vi "Close PDF refnum.vi"(1 "Data IN":T1={"Document"=refnum, "Writer"=refnum, "Default Font"=refnum, "Default Font cluster"={"Name"="Helvetica", "Size"=12.0, "Color"=0, "Style"={"Bold"=FALSE, "Italic"=FALSE, "Underline"=FALSE, "Strikeout"=FALSE}}, "Path"=path "", "Unit (default = mm)"=enum."mm", "Paragraphe cluster"={" Aligment"=enum."Select", "Line spacing"=enum."Select"}, "Pages dimensions [ ]"=[], "Captions"={"Image"={"Caption"="", "Separator"="", "Position"=enum."Above"}, "Image counter"=0, "Table"={"Caption"="", "Separator"="", "Position"=enum."Above"}, "Table counter"=0, "Font"={"Name"="", "Size"=-1.0, "Color"=0, "Style"={"Bold"=FALSE, "Italic"=FALSE, "Underline"=FALSE, "Strikeout"=FALSE}}}, "Header"=[], "Footer"=[], "Watermark "={"Show? (F)"=FALSE, "Type"=enum."Text", "Opacity (%)"=10.0, "Rotate(°)"=0.0, "Position"={"Position"=enum."Center (text section)", "X"=0.0, "Y"=0.0}, "Image path"=path "", "Scaled(%)"=100.0, "Image refnum"=refnum, "Text"="CONFIDENTIAL", "Font"={"Name"="", "Size"=-1.0, "Color"=0}, "Font refnum"=refnum, "Alignment"=enum."Center", "Automatic"=FALSE}, "Actual VI name"="", "System Fonts"={"Font name [ ]"=[], "Font and file names [ ]"=[]}} caption="Data") -> (0 "Data OUT":T1={"Document"=refnum, "Writer"=refnum, "Default Font"=refnum, "Default Font cluster"={"Name"="Helvetica", "Size"=12.0, "Color"=0, "Style"={"Bold"=FALSE, "Italic"=FALSE, "Underline"=FALSE, "Strikeout"=FALSE}}, "Path"=path "", "Unit (default = mm)"=enum."mm", "Paragraphe cluster"={" Aligment"=enum."Select", "Line spacing"=enum."Select"}, "Pages dimensions [ ]"=[], "Captions"={"Image"={"Caption"="", "Separator"="", "Position"=enum."Above"}, "Image counter"=0, "Table"={"Caption"="", "Separator"="", "Position"=enum."Above"}, "Table counter"=0, "Font"={"Name"="", "Size"=-1.0, "Color"=0, "Style"={"Bold"=FALSE, "Italic"=FALSE, "Underline"=FALSE, "Strikeout"=FALSE}}}, "Header"=[], "Footer"=[], "Watermark "={"Show? (F)"=FALSE, "Type"=enum."Text", "Opacity (%)"=10.0, "Rotate(°)"=0.0, "Position"={"Position"=enum."Center (text section)", "X"=0.0, "Y"=0.0}, "Image path"=path "", "Scaled(%)"=100.0, "Image refnum"=refnum, "Text"="CONFIDENTIAL", "Font"={"Name"="", "Size"=-1.0, "Color"=0}, "Font refnum"=refnum, "Alignment"=enum."Center", "Automatic"=FALSE}, "Actual VI name"="", "System Fonts"={"Font name [ ]"=[], "Font and file names [ ]"=[]}} caption="Data")   [LabVIEW 2012]
uses:
  PDF Report Data.ctl
  C:/Users/MaxCorp/Documents/TopPerm - Base/DLL/itextsharp.dll
  DLL/itextsharp.dll
  Font cluster.ctl
  Font size.ctl
  Font color.ctl
  Unit.ctl
  Paragraphe cluster.ctl
  Texte alignement.ctl
  Line spacing.ctl
  Page dimensions.ctl
  Page Orientation.ctl
  Image or Table Caption.ctl
  Header Footer [ ].ctl
  Header Footer cluster.ctl
  Header Footer Type.ctl
  Header footer horiz alignment.ctl
  Cell Vertical alignment.ctl
  Page number.ctl
  Header Footer Line.ctl
  Watermark cluster2.ctl
  Watermark Position.ctl
  System Fonts.ctl
  PDF Report.xctl
panel:
  # "X"
  # "Y"
  # "X"
  # "Y"
  # "X"
  # "Y"
  # "X"
  # "Y"
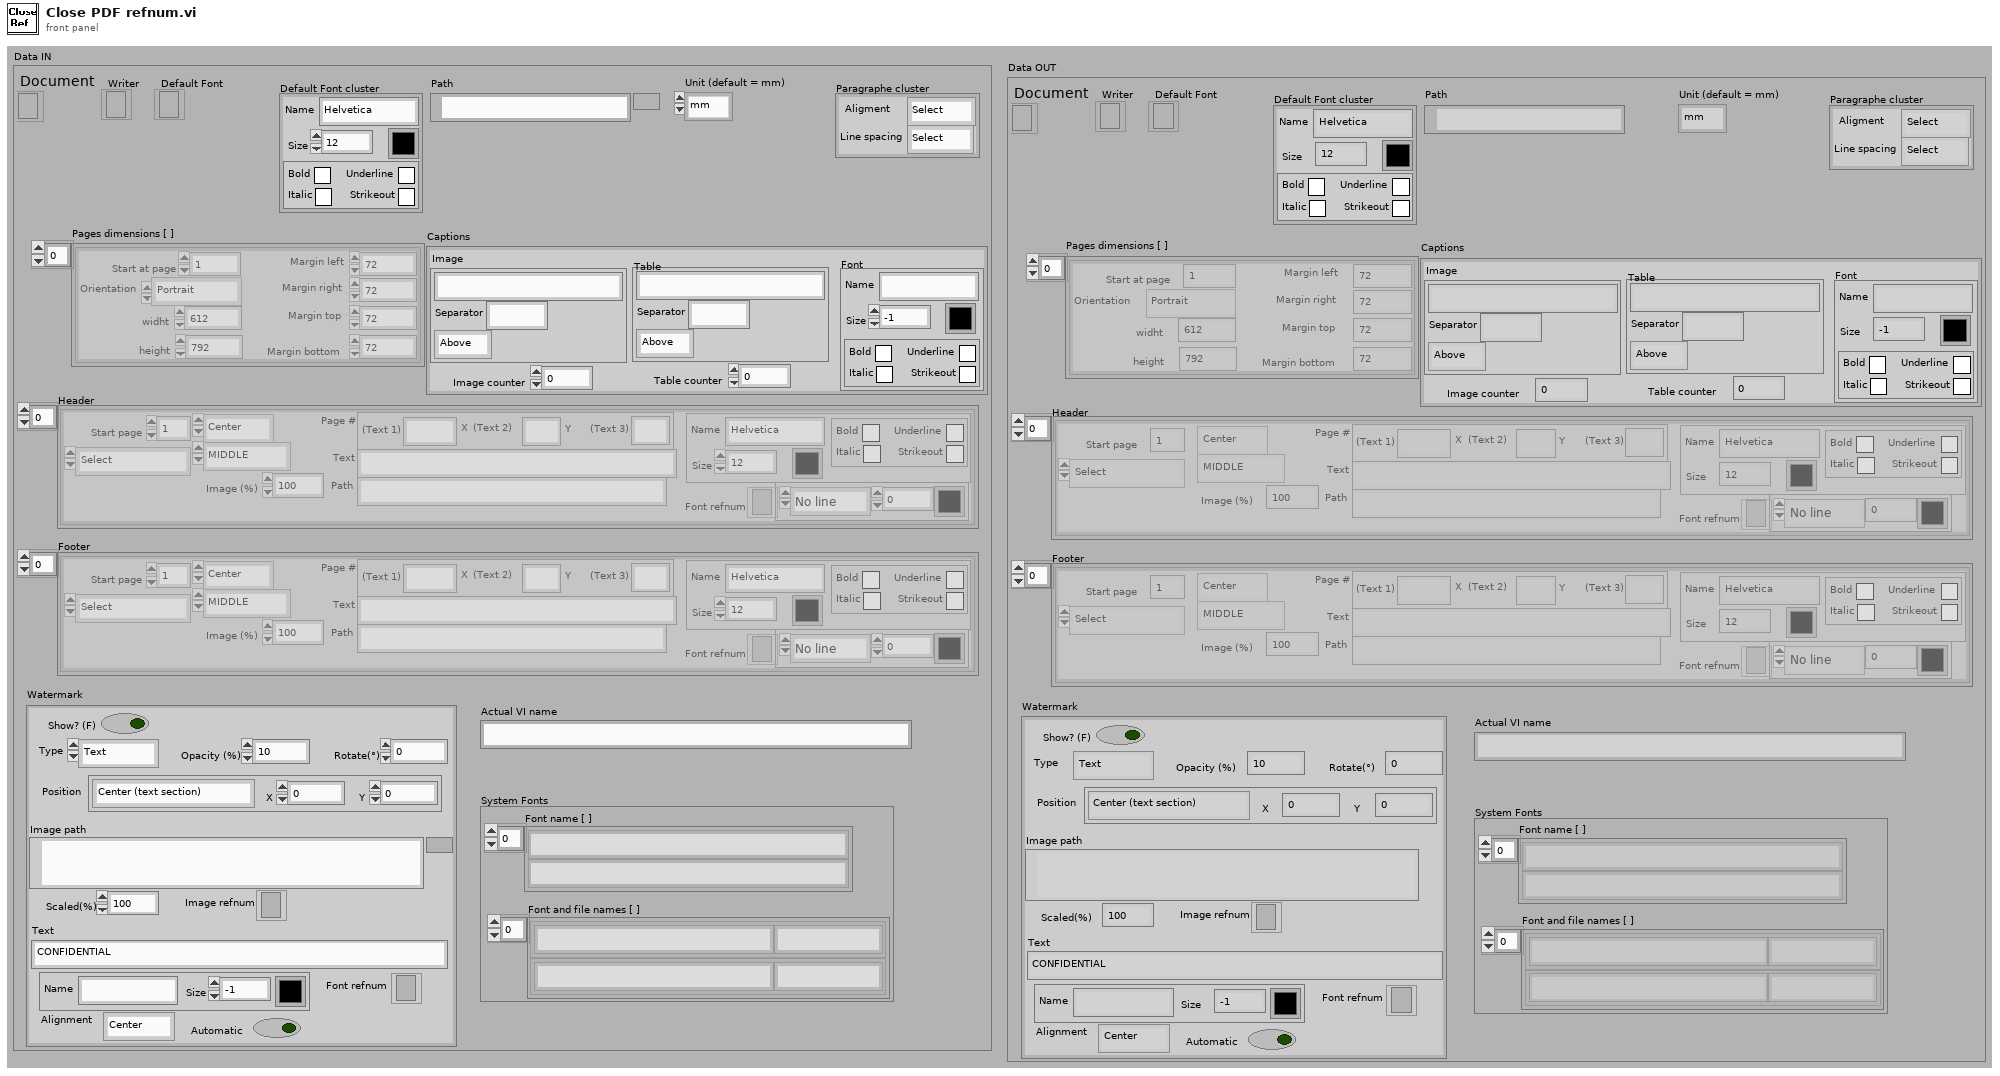
[diagram p1: front panel]
types:
  T1 = typedef "PDF Report.xctl/PDF Report Data.ctl" = cluster{"Document":refnum<k24>, "Writer":refnum<k24>, "Default Font":refnum<k24>, "Default Font cluster":T2, "Path":path, "Unit (default = mm)":T5, "Paragraphe cluster":T6, "Pages dimensions [ ]":T9[], "Captions":cluster{"Image":T11, "Image counter":u16, "Table":T11, "Table counter":u16, "Font":T2}, "Header":T12, "Footer":T12, "Watermark ":T19, "Actual VI name":string, "System Fonts":T21}
  T2 = typedef "Font cluster.ctl" = cluster{"Name":string, "Size":T3, "Color":T4, "Style":cluster{"Bold":bool, "Italic":bool, "Underline":bool, "Strikeout":bool}}
  T3 = typedef "Font size.ctl" = sgl
  T4 = typedef "Font color.ctl" = u32
  T5 = typedef "Unit.ctl" = enum16{"inch", "mm"}
  T6 = typedef "Paragraphe cluster.ctl" = cluster{" Aligment":T7, "Line spacing":T8}
  T7 = typedef "Texte alignement.ctl" = enum16{"Select", "CENTER", "JUSTIFY", "LEFT", "RIGHT"}
  T8 = typedef "Line spacing.ctl" = enum16{"Select", "1.0", "1.5", "2.0"}
  T9 = typedef "Page dimensions.ctl" = cluster{"Start at page":i32, "Orientation":T10, "widht":sgl, "height":sgl, "Margin left":sgl, "Margin right":sgl, "Margin top":sgl, "Margin bottom":sgl}
  T10 = typedef "Page Orientation.ctl" = enum16{"Portrait", "Landscape"}
  T11 = typedef "Image or Table Caption.ctl" = cluster{"Caption":string, "Separator":string, "Position":enum16{"Above", "Below"}}
  T12 = typedef "Header Footer [ ].ctl" = T13[]
  T13 = typedef "Header Footer cluster.ctl" = cluster{"Start page":i32, "Type":T14, "Alignment":T15, "Vertical Alignement":T16, "Image (%)":sgl, "Page #":T17, "Text":string, "Path":string, "Font":T2, "Font refnum":refnum<k24>, "Line":cluster{"Line":T18, "Thickness (points)":sgl, "Colour":T4}}
  T14 = typedef "Header Footer Type.ctl" = enum16{"Select", "Text", "Text + hyperlink", "Page number", "Image", "Image + hyperlink"}
  T15 = typedef "Header footer horiz alignment.ctl" = enum16{"Left", "Center", "Right"}
  T16 = typedef "Cell Vertical alignment.ctl" = enum16{"TOP", "MIDDLE", "BOTTOM"}
  T17 = typedef "Page number.ctl" = cluster{"Text 1":string, "Text 2":string, "Text 3":string}
  T18 = typedef "Header Footer Line.ctl" = enum16{"No line", "Horizontal line"}
  T19 = typedef "Watermark cluster2.ctl" = cluster{"Show? (F)":bool, "Type":enum16{"Image", "Text"}, "Opacity (%)":sgl, "Rotate(°)":sgl, "Position":cluster{"Position":T20, "X":sgl, "Y":sgl}, "Image path":path, "Scaled(%)":sgl, "Image refnum":refnum<k24>, "Text":string, "Font":cluster{"Name":string, "Size":T3, "Color":T4}, "Font refnum":refnum<k24>, "Alignment":T15, "Automatic":bool}
  T20 = typedef "Watermark Position.ctl" = enum16{"Absolute", "Center (page)", "Center (text section)"}
  T21 = typedef "System Fonts.ctl" = cluster{"Font name [ ]":string[], "Font and file names [ ]":cluster{"Font name":string, "File name":string}[]}
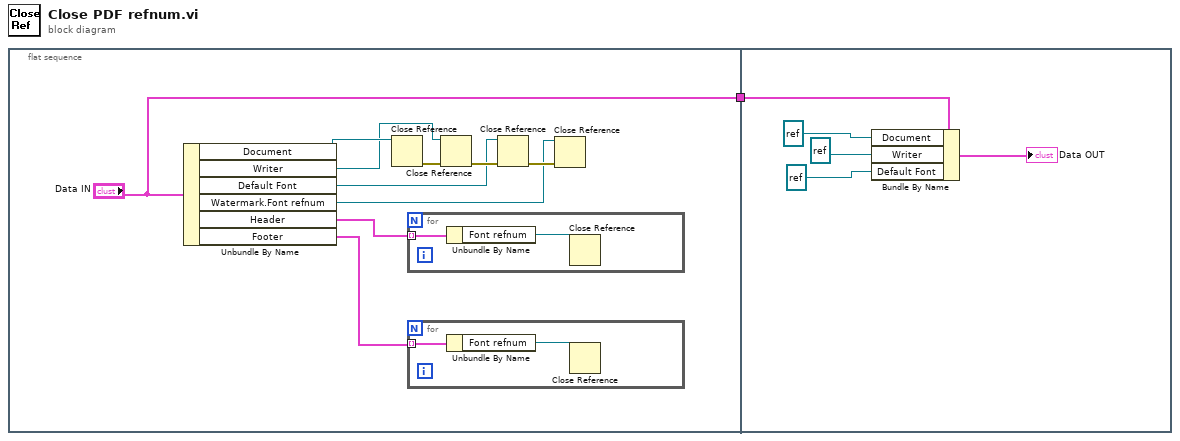
[diagram p0: block diagram]
diagram:
  n1 = flat-sequence {
    tunnel: ["Data IN"] -> w1
    tunnel: w1 -> [w16]
    frame #0 {
      n2 = Unbundle By Name("Data IN") -> ("Document"=w10:refnum<k24>, "Writer"=w7:refnum<k24>, "Default Font"=w9:refnum<k24>, "Watermark.Font refnum"=w4:refnum<k24>, "Header"=w3:T12, "Footer"=w2:T12)
      n3 = Close Reference(reference=w10) -> (error out=w8:errorcluster)  [unwired: 1 in]
      n4 = for {
        tunnel: w3 -> [w15] mode=indexing
        n5 = Unbundle By Name(w15) -> ("Font refnum"=w14:refnum<k24>)
        n6 = Close Reference(reference=w14) -> ()  [unwired: 1 in, 1 out]
      }
      n7 = for {
        tunnel: w2 -> [w13] mode=indexing
        n8 = Unbundle By Name(w13) -> ("Font refnum"=w12:refnum<k24>)
        n9 = Close Reference(reference=w12) -> ()  [unwired: 1 in, 1 out]
      }
      n10 = Close Reference(reference=w7, error in (no error)=w8) -> (error out=w11:errorcluster)
      n11 = Close Reference(reference=w9, error in (no error)=w11) -> (error out=w5:errorcluster)
      n12 = Close Reference(reference=w4, error in (no error)=w5) -> ()  [unwired: 1 out]
    }
    frame #1 {
      n13 = Bundle By Name(cluster=w16, "Document"=refnum<k24> refnum, "Writer"=refnum<k24> refnum, "Default Font"=refnum<k24> refnum ("Font")) -> (→"Data OUT":T1)
    }
  }
